vi "E2.vi"() -> ()   [LabVIEW 2018]
uses:
  Control 4.ctl
  Control 2.ctl
  Control 3.ctl
  Control 1.ctl
panel:
  in  "Numeric":T1
  out "Binary phase shift":dbl[](graph)
  out "Modulating signal":dbl[](graph)
  in  "Modulating freq":T2
  in  "Sampling freq":T3
  in  "Carrier freq":T4
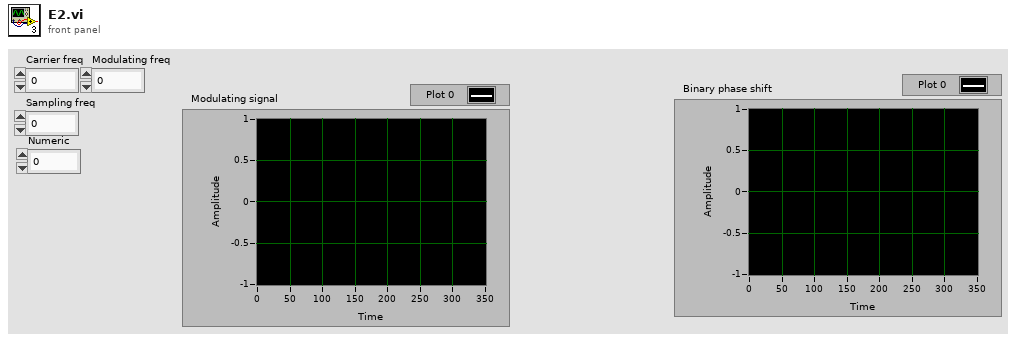
[diagram p1: front panel]
types:
  T1 = typedef "Control 1" = i32
  T2 = typedef "Control 3" = dbl
  T3 = typedef "Control 2" = dbl
  T4 = typedef "Control 4" = dbl
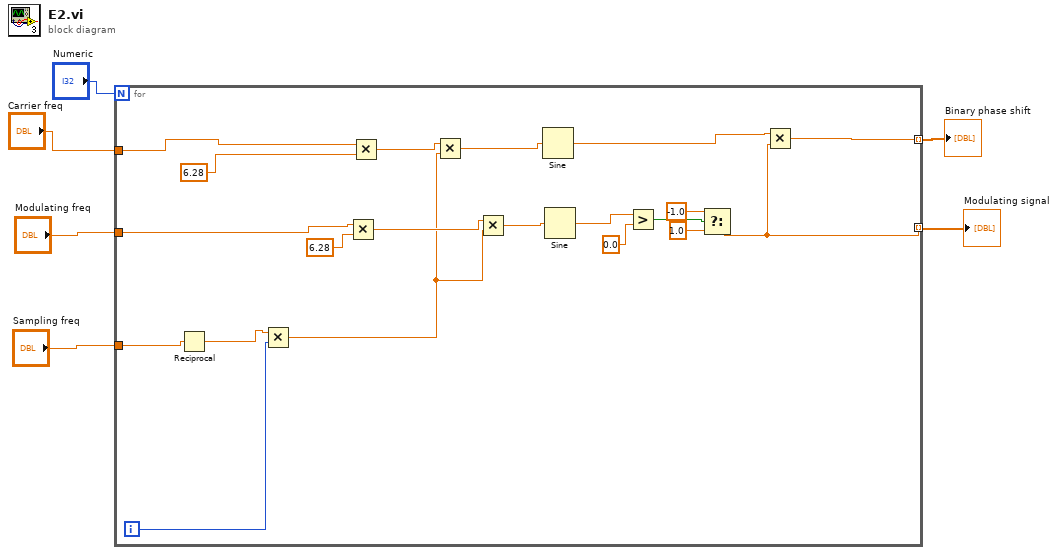
[diagram p0: block diagram]
diagram:
  n1 = for {
    N: "Numeric" -> [_]
    tunnel: "Carrier freq" -> [w25]
    tunnel: "Sampling freq" -> [w24]
    tunnel: "Modulating freq" -> [w20]
    tunnel: [w8] -> w3 mode=indexing
    tunnel: [w7] -> w2 mode=indexing
    i -> [w22]
    n2 = Reciprocal(x=w24) -> (1/x=w23:T3)
    n3 = Multiply(x=w23, y=w22) -> (x*y=w17:T3)
    n4 = Multiply(x=w20, y=6.28) -> (x*y=w18:T2)
    n5 = Multiply(x=w25, y=6.28) -> (x*y=w21:T4)
    n6 = Multiply(x=w21, y=w17) -> (x*y=w16:T4)
    n7 = Multiply(x=w18, y=w17) -> (x*y=w15:T2)
    n8 = Sine(x=w16) -> (sin(x)=w9:T4)
    n9 = Sine(x=w15) -> (sin(x)=w14:T2)
    n10 = Greater?(x=w14, y=0.0) -> (0:w12:bool)
    n11 = Select(t=-1.0, s=w12, f=1.0) -> (s? t:f=w7:dbl)
    n12 = Multiply(x=w9, y=w7) -> (x*y=w8:T4)
  }
  "Binary phase shift" <- w3
  "Modulating signal" <- w2
